vi "globala.vi"() -> ()   [LabVIEW 2015]
panel:
  out "Numeric":dbl
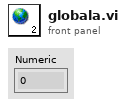
[diagram p1: front panel]
diagram:
